vi "Shut_Down_Client_Demands.vi"(1 "Ch Names":string[](array[string]), 2 "Values":dbl[](array[numeric]) format="%.2f", 3 "Client Name":string) -> (0 "Comments":string)   [LabVIEW 2010]
uses:
  ADAM_Global.vi
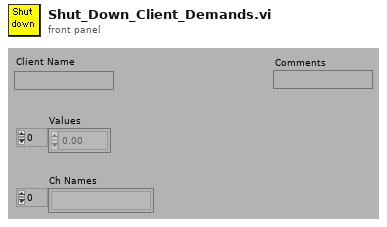
[diagram p1: front panel]
types:
  T1 = typedef "Server_Control.ctl" = cluster{"Channel Name to control":string, "Channel sharing":enum16{"Channel Unshared", "Channel Shared by Rig", "Channel Shared by Group"}, "Default Value":dbl, "Client Array":string[], "Time Stamp":timestamp, "Do Not Reset":bool}
  T2 = enum16{"Channel Unshared", "Channel Shared by Rig", "Channel Shared by Group"}
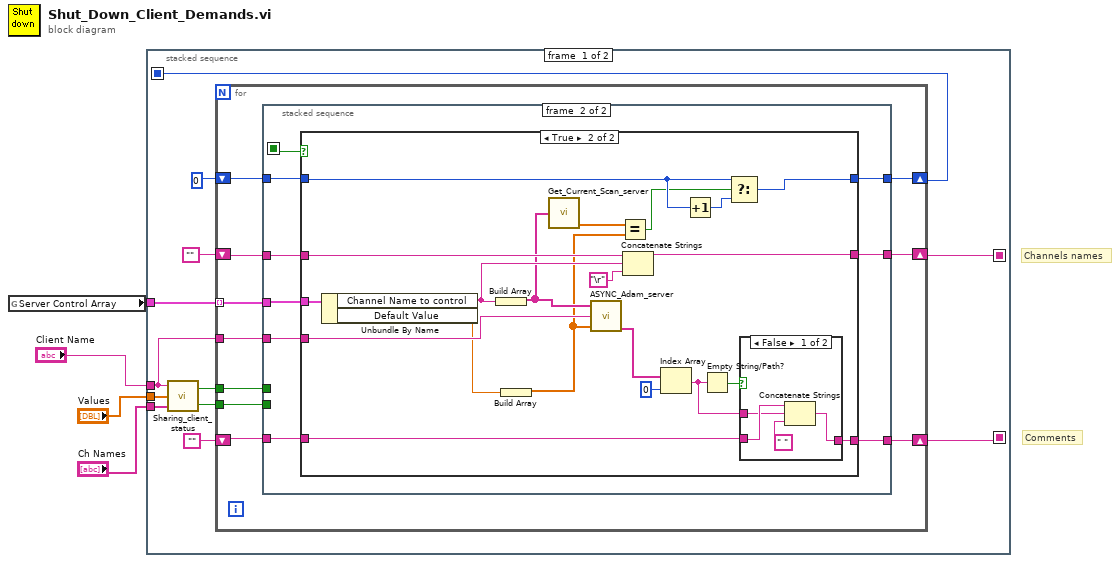
[diagram p0: block diagram]
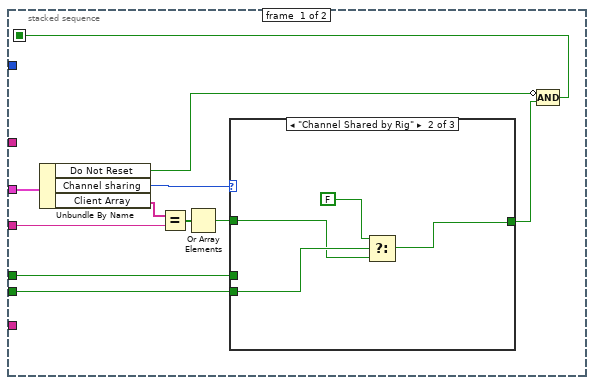
[diagram p2: hidden frame]
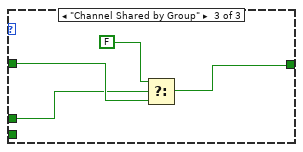
[diagram p4: hidden frame]
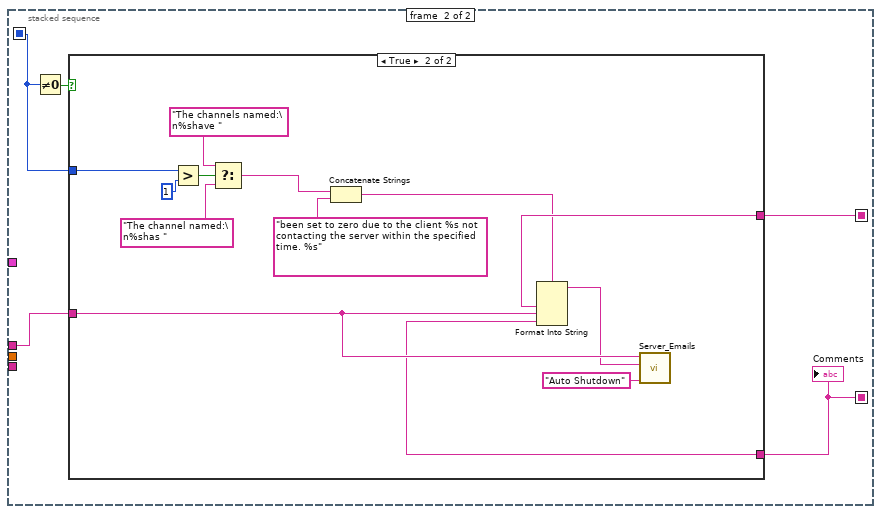
[diagram p7: hidden frame]
diagram:
  # "Channels names"
  # "Comments"
  n1 = global read "ADAM_Global.vi" "Server Control Array"() -> (w4:T1[])
  n2 = stacked-sequence {
    seq-local: [w8 _] -> [_ w87]
    seq-local: [w9 _] -> [_ w84]
    seq-local: [w7 _] -> [_ w86]
    tunnel: w4 -> [w16 _]
    tunnel: "Client Name" -> [w10 w85]
    tunnel: "Values" -> [w6 _]
    tunnel: "Ch Names" -> [w5 _]
    frame #0 {
      n3 = call "Sharing_client_status.vi"("Ch Names"=w5, "Values"=w6, "Client Name"=w10) -> ("Active Machines in Rig"=w15:bool, "Active Machines in Group"=w14:bool)
      n4 = for {
        tunnel: w16 -> [w26] mode=indexing
        tunnel: w10 -> [w25]
        tunnel: w15 -> [w24]
        tunnel: w14 -> [w23]
        shift-right: [w21] -> w9
        shift-left: "" -> [w22]
        shift-right: [w19] -> w7
        shift-left: "" -> [w20]
        shift-right: [w17] -> w8
        shift-left: 0 -> [w18]
        n5 = stacked-sequence {
          seq-local: [w27 _] -> [_ w55]
          tunnel: w26 -> [w37 w54]
          tunnel: w25 -> [w34 w53]
          tunnel: w24 -> [w32 _]
          tunnel: w23 -> [w31 _]
          tunnel: w22 -> [_ w52]
          tunnel: [_ w51] -> w21
          tunnel: w20 -> [_ w50]
          tunnel: [_ w49] -> w19
          tunnel: w18 -> [_ w48]
          tunnel: [_ w47] -> w17
          frame #0 {
            n6 = Unbundle By Name(w37) -> ("Do Not Reset"=w28:bool, "Channel sharing"=w36:T2, "Client Array"=w35:string[])
            n7 = Equal?(x=w35, y=w34) -> (x = y?=w33:bool[])
            n8 = Or Array Elements(Boolean array=w33) -> (logical OR=w30:bool)
            n9 = case shown="\"Channel Shared by Rig\"" w36 {
              tunnel: [w38 w39 w44] -> w29
              tunnel: w30 -> [w38 w41 w46]
              tunnel: w32 -> [_ w42 _]
              tunnel: w31 -> [_ _ w43]
              frame "Channel Unshared" {
              }
              frame "Channel Shared by Rig" {
                n10 = Select(t=FALSE, s=w42, f=w41) -> (s? t:f=w39:bool)
              }
              frame "Channel Shared by Group" {
                n11 = Select(t=FALSE, s=w43, f=w46) -> (s? t:f=w44:bool)
              }
            }
            n12 = Compound Arithmetic op=AND(invert w28, w29) -> (w27:bool)
          }
          frame #1 {
            n13 = case shown="True" w55 {
              tunnel: w54 -> [_ w78]
              tunnel: w53 -> [_ w71]
              tunnel: w52 -> [w58 w75]
              tunnel: [w58 w74] -> w51
              tunnel: w50 -> [w56 w70]
              tunnel: [w56 w69] -> w49
              tunnel: w48 -> [w57 w62]
              tunnel: [w57 w63] -> w47
              frame False {
              }
              frame True {
                n14 = Unbundle By Name(w78) -> ("Channel Name to control"=w68:string, "Default Value"=w67:dbl)
                n15 = Build Array(w68) -> (w66:string[])
                n16 = Build Array(w67) -> (w64:dbl[])
                n17 = call "Get_Current_Scan_server.vi"("Desired Channels"=w66) -> ("Numerical Values"=w65:dbl[])  [unwired: 2 out]
                n18 = call "ASYNC_Adam_server.vi"("Values"=w64, "Client Name"=w71, "Channel Names"=w66) -> ("Scan Comments"=w77:string[])  [unwired: 2 out]
                n19 = Equal?(x=w65, y=w64) -> (x = y?=w60:bool)
                n20 = Concatenate Strings(w70, w68, "\r") -> (w69:string)
                n21 = Index Array(array=w77, index=0 ("Index")) -> (element=w72:string)
                n22 = Increment(x=w62) -> (x+1=w61:i32)
                n23 = Empty String/Path?(string/path=w72) -> (empty?=w73:bool)
                n24 = Select(t=w62, s=w60, f=w61) -> (s? t:f=w63:i32)
                n25 = case shown="False" w73 {
                  tunnel: w75 -> [w81 w83]
                  tunnel: [w82 w83] -> w74
                  tunnel: w72 -> [w80 _]
                  frame False {
                    n26 = Concatenate Strings(w81, w80, " ") -> (w82:string)
                  }
                  frame True {
                  }
                }
              }
            }
          }
        }
      }
    }
    frame #1 {
      n27 = Not Equal To 0?(x=w87) -> (x != 0?=w88:bool)
      n28 = case shown="True" w88 {
        tunnel: w87 -> [_ w101]
        tunnel: w86 -> [_ w100]
        tunnel: w85 -> [_ w99]
        tunnel: w84 -> [_ w98]
        frame False {
        }
        frame True {
          n29 = Greater?(x=w101, y=1) -> (0:w95:bool)
          n30 = Select(t="The channels named:\n%shave ", s=w95, f="The channel named:\n%shas ") -> (s? t:f=w93:string)
          n31 = Concatenate Strings(w93, "been set to zero due to the client %s not contacting the server within the specified time. %s" ("Substring")) -> (w91:string)
          n32 = Format Into String(format string=w91, w100, w99, w98) -> (resulting string=w90:string)  [unwired: 2 in, 1 out]
          n33 = call "Server_Emails.vi"("Client Name Contains"=w99, "Message"=w90, "Subject"="Auto Shutdown") -> ()  [unwired: 2 in, 3 out]
        }
      }
      "Comments" <- w84
    }
  }
